vi "test multi mag orbit derivatives.vi"() -> ()   [LabVIEW 2017]
uses:
  typedefs/orbit parameters full.ctl
  typedefs/magnetomter reading set.ctl
panel:
  out "rel diff":dbl[][](array[numeric]) format="%#_1e"
  out "abs difference":dbl[][](array[numeric]) format="%#_2p"
  out "size(s) 2":i32[](array[numeric])
  out "size(s)":i32[](array[numeric])
  out "derivatives":dbl[][](array[numeric]) format="%#_2p"
  out "numeric derivatives":dbl[][](array[numeric]) format="%#_2p"
  in  "orbit parameters":T1={"a"=75.0, "b"=0.0, "theta_axis"=0.0, "dPhi"=0.09695731996962338, "BrV"=-990.802948176856, "bob tilt"=0.29876226934427874, "phi0"=6.999694380286486, "phi_dot"=-6.2, "x0"=0.0, "y0"=0.0, "z0"=54.40192502595471}
  # "dphi"
  # "b"
  # "th"
  # "a"
  # "phi0"
  # "phidot"
  # "z0"
  # "x0"
  # "brv"
  # "bob tilt"
  # "y0"
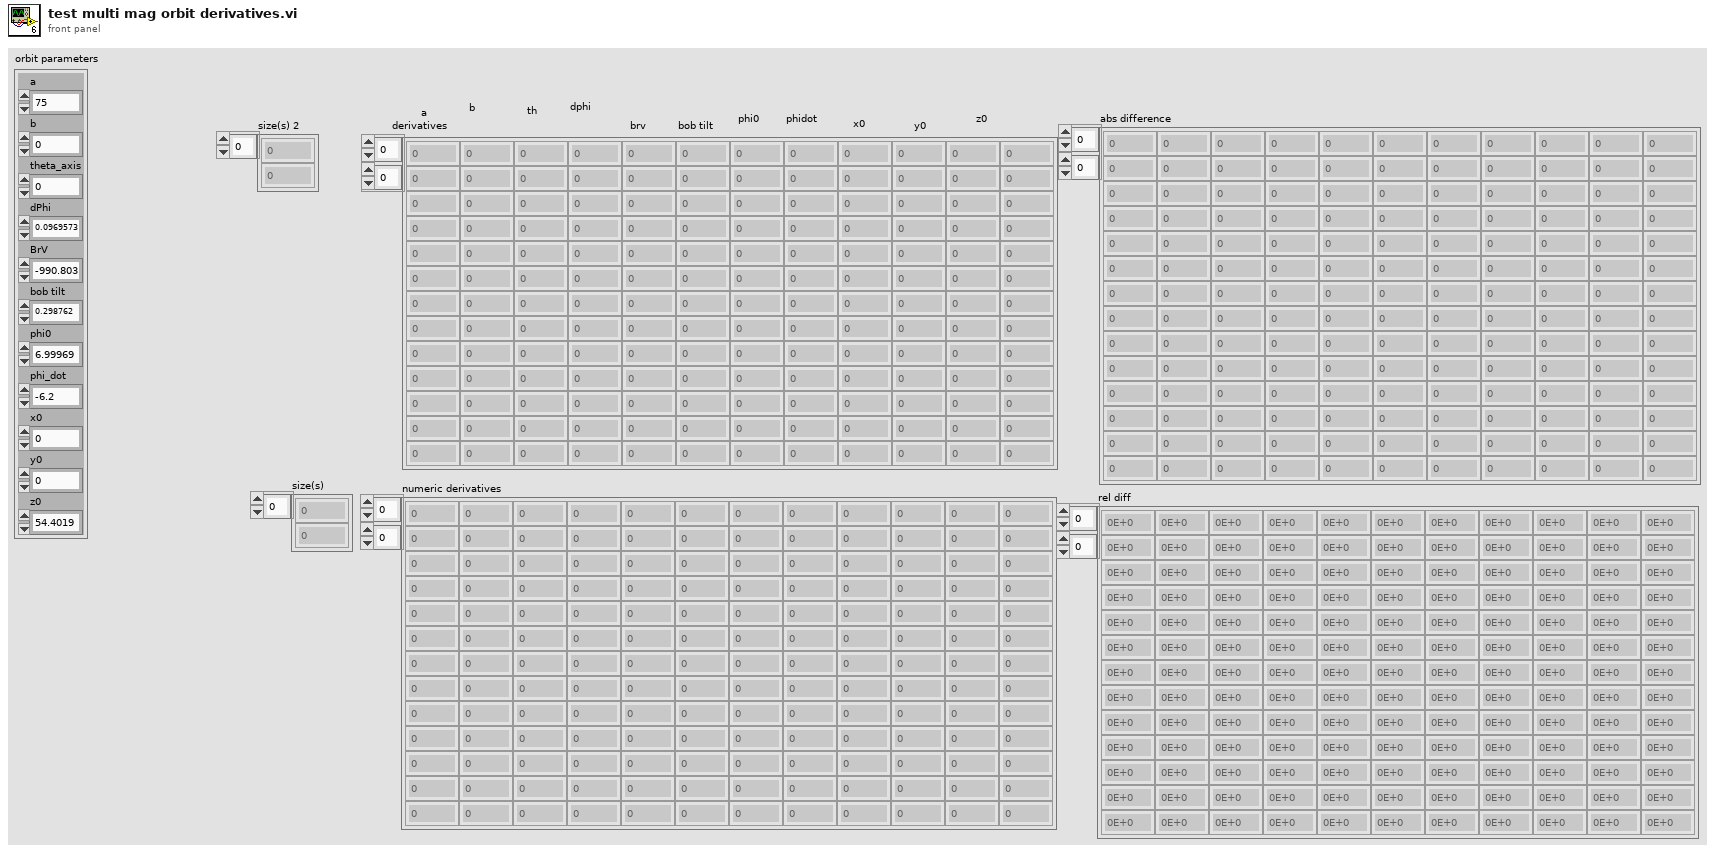
[diagram p1: front panel]
types:
  T1 = typedef "orbit parameters full.ctl" = cluster{"a":dbl, "b":dbl, "theta_axis":dbl, "dPhi":dbl, "BrV":dbl, "bob tilt":dbl, "phi0":dbl, "phi_dot":dbl, "x0":dbl, "y0":dbl, "z0":dbl}
  T2 = typedef "magnetomter reading set.ctl" = cluster{"time":fxp<+,48,48>, "mag readings":cluster{"magnetometer index":dbl, "Bx":dbl, "By":dbl, "Bz":dbl, "magnetometer x":dbl, "magnetometer y":dbl}[]}
  T3 = cluster{"orbit parameters[0]":dbl, "orbit parameters[1]":dbl, "orbit parameters[2]":dbl, "orbit parameters[3]":dbl, "orbit parameters[4]":dbl, "orbit parameters[5]":dbl, "orbit parameters[6]":dbl, "orbit parameters[7]":dbl, "orbit parameters[8]":dbl, "orbit parameters[9]":dbl, "orbit parameters[10]":dbl}
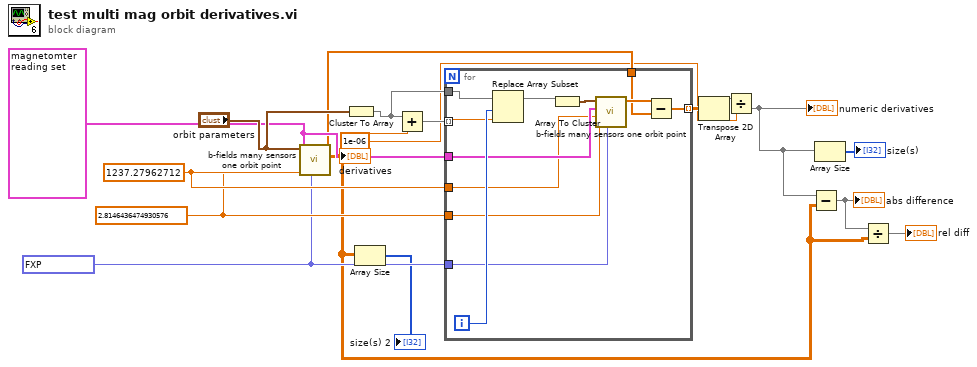
[diagram p0: block diagram]
diagram:
  w8 = 1e-06 ("y")
  w11 = fxp<+,48,48> 18870679552.0 ("t0")
  w14 = T2 {"time"=18872893554.0, "mag readings"=[{"magnetometer index"=0.0, "Bx"=-172.0634765625, "By"=-2.54296875, "Bz"=-1428.453125, "magnetometer x"=0.0, "magnetometer y"=0.0}, {"magnetometer index"=1.0, "Bx"=-208.375, "By"=357.4306640625, "Bz"=-182.794921875, "magnetometer x"=-22.5, "magnetometer y"=38.971}, {"magnetometer index"=2.0, "Bx"=-210.4453125, "By"=-333.25390625, "Bz"=-193.001953125, "magnetometer x"=-22.5, "magnetometer y"=-38.971}, {"magnetometer index"=3.0, "Bx"=467.15234375, "By"=36.216796875, "Bz"=-244.134765625, "magnetometer x"=45.0, "magnetometer y"=0.0}]} ("magnetometer readings")
  w12 = 2.8146436474930576 ("omega")
  w13 = 1237.27962712 ("L")
  n1 = call "b-fields many sensors one orbit point.vi"("t0"=w11, "omega"=w12, "L"=w13, "magnetometer readings"=w14, "orbit parameters"="orbit parameters") -> ("derivatives"=w2:dbl[][], "predicted field"=w10:dbl[])  [unwired: 1 in, 4 out]
  "derivatives" <- w2
  n2 = Cluster To Array(cluster="orbit parameters") -> (array=w15:dbl[])
  n3 = Array Size(array=w2) -> (size(s)=→"size(s) 2":i32[])
  n4 = Add(x=w15, y=w8) -> (x+y=w16:dbl[])
  n5 = for {
    tunnel: w16 -> [w27] mode=indexing
    tunnel: w15 -> [w29]
    tunnel: w14 -> [w24]
    tunnel: w13 -> [w23]
    tunnel: w12 -> [w22]
    tunnel: w11 -> [w21]
    tunnel: w10 -> [w19]
    tunnel: [w18] -> w9 mode=indexing
    i -> [w28]
    n6 = Replace Array Subset(array=w29, new element=w27, index=w28) -> (w26:dbl[])
    n7 = Array To Cluster(array=w26) -> (cluster=w25:T3)
    n8 = call "b-fields many sensors one orbit point.vi"("t0"=w21, "omega"=w22, "L"=w23, "magnetometer readings"=w24, "orbit parameters"=w25) -> ("predicted field"=w20:dbl[])  [unwired: 1 in, 5 out]
    n9 = Subtract(x=w20, y=w19) -> (x-y=w18:dbl[])
  }
  n10 = Transpose 2D Array(2D array=w9) -> (transposed array=w5:dbl[][])
  n11 = Divide(x=w5, y=w8) -> (x/y=w4:dbl[][])
  "numeric derivatives" <- w4
  n12 = Subtract(x=w4, y=w2) -> (x-y=w3:dbl[][])
  "abs difference" <- w3
  n13 = Array Size(array=w4) -> (size(s)=→"size(s)":i32[])
  n14 = Divide(x=w3, y=w2) -> (x/y=→"rel diff":dbl[][])
